vi "Sequence.GetVersion.vi"(8 "error in (no error)":errorcluster, 10 "Exists":bool, 11 "Path":path) -> (0 "error out":errorcluster, 3 "Build":u32)   [LabVIEW 2015, in "Simple Sequence Tools - Shared.lvlib"]
uses:
  Simple Sequence Tools - Shared.lvlib
  NationalInstruments.VeriStand.RealTimeSequenceDefinitionApi
  NationalInstruments.VeriStand
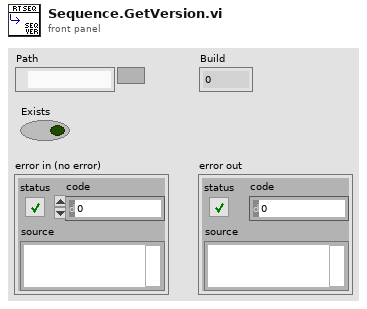
[diagram p1: front panel]
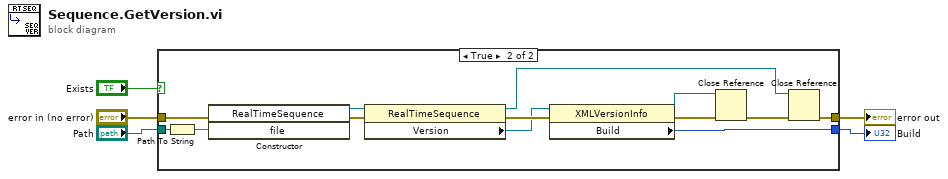
[diagram p0: block diagram]
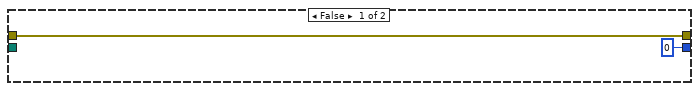
[diagram p2: hidden frame]
diagram:
  n1 = case shown="True" "Exists" {
    tunnel: "Path" -> [_ w11]
    tunnel: "error in (no error)" -> [w6 w10]
    tunnel: [w6 w9] -> w3
    tunnel: [u32 0 ("Build") w8] -> w5
    frame False {
    }
    frame True {
      n2 = Path To String(path=w11) -> (string=w12:string)
      n3 = constructor class="RealTimeSequence"(error in=w10, "file"=w12) -> (reference out=w20:refnum<k24>, error out=w19:errorcluster)  [unwired: 2 in, 2 out]
      n4 = property class="RealTimeSequence"(reference=w20, error in=w19) -> (reference out=w14:refnum<k24>, error out=w18:errorcluster, "Version"=w17:refnum<k24>)
      n5 = property class="XMLVersionInfo"(reference=w17, error in=w18) -> (reference out=w15:refnum<k24>, error out=w16:errorcluster, "Build"=w8:u32)
      n6 = Close Reference(reference=w15, error in (no error)=w16) -> (error out=w13:errorcluster)
      n7 = Close Reference(reference=w14, error in (no error)=w13) -> (error out=w9:errorcluster)
    }
  }
  "Build" <- w5
  "error out" <- w3
